vi "niFpgaBFGroupLastEven.vi"(5 "bf data in":T1 {"x_r" format="%.16g"; "x_i" format="%.16g"; "y_r" format="%.16g"; "y_i" format="%.16g"}, 7 "stage switch in":bool, 9 "tf index in":fxp<+,7,7>) -> (6 "bf data out":T1 {"x_r" format="%.16g"; "x_i" format="%.16g"; "y_r" format="%.16g"; "y_i" format="%.16g"}, 8 "stage switch out":bool)   [LabVIEW 2017]
uses:
  <vilib>/rvi/FXPMathLib/basic elements/FxpDiscreteDelay/XNode/nifxpmath_DiscreteDelay.xnode
  <vilib>/rvi/Analysis/measure/FFT/supportingXNodes/permutation/XNode/niFpgaFFTPermutation.xnode
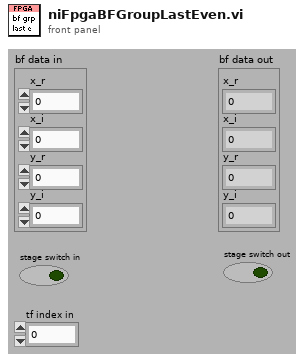
[diagram p1: front panel]
types:
  T1 = cluster{"x_r":fxp<+/-,16,1>, "x_i ":fxp<+/-,16,1>, "y_r ":fxp<+/-,16,1>, "y_i ":fxp<+/-,16,1>}
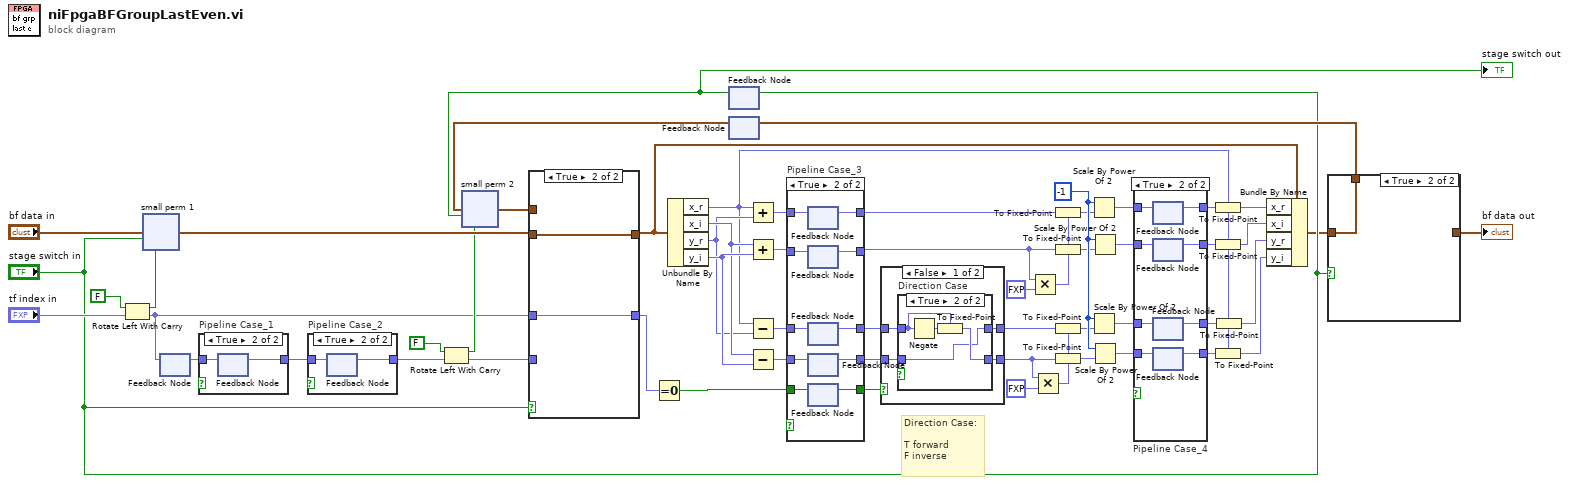
[diagram p0: block diagram]
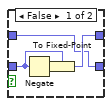
[diagram p6: hidden frame]
diagram:
  w31 = -1 ("n")
  # "Direction Case:\n\nT forward\nF inverse"
  n1 = Rotate Left With Carry(2:"tf index in", 3:FALSE ("carry")) -> (0:w34:fxp<+,7,7>, 1:w50:bool)
  n2 = xnode "small perm 1"("bf data in"="bf data in", "stage switch"="stage switch in", "perm switch"=w50) -> ("bf data out"=w49:T1)
  n3 = feedback-in #1(w34) -> ()
  n4 = feedback #1() -> (w11:fxp<+,7,7>)  [unwired: 1 in]
  n5 = case "Pipeline Case_1" shown="True" {
    selector: _ -> [_ _]
    tunnel: w11 -> [w59 w61]
    tunnel: [w59 w60] -> w2
    frame False {
    }
    frame True {
      n6 = feedback-in #2(w61) -> ()
      n7 = feedback #2() -> (w60:fxp<+,7,7>)  [unwired: 1 in]
    }
  }
  n8 = case "Pipeline Case_2" shown="True" {
    selector: _ -> [_ _]
    tunnel: w2 -> [w62 w64]
    tunnel: [w62 w63] -> w1
    frame False {
    }
    frame True {
      n9 = feedback-in #3(w64) -> ()
      n10 = feedback #3() -> (w63:fxp<+,7,7>)  [unwired: 1 in]
    }
  }
  n11 = Rotate Left With Carry(2:w1, 3:FALSE ("carry")) -> (0:w53:fxp<+,7,7>, 1:w48:bool)
  n12 = feedback-in #4("stage switch in") -> ()
  n13 = feedback #4() -> (w45:bool)  [unwired: 1 in]
  "stage switch out" <- w45
  n14 = feedback #5() -> (w47:T1)  [unwired: 1 in]
  n15 = xnode "small perm 2"("bf data in"=w47, "stage switch"=w45, "perm switch"=w48) -> ("bf data out"=w46:T1)
  n16 = case shown="True" "stage switch in" {
    tunnel: [w66 w68] -> w37
    tunnel: w49 -> [_ w68]
    tunnel: w46 -> [w66 _]
    tunnel: w53 -> [w65 _]
    tunnel: [w65 w67] -> w26
    tunnel: w34 -> [_ w67]
    frame False {
    }
    frame True {
    }
  }
  n17 = Equal To 0?(x=w26) -> (x = 0?=w13:bool)
  n18 = Unbundle By Name(w37) -> ("x_r"=w35:fxp<+/-,16,1>, "x_i"=w41:fxp<+/-,16,1>, "y_r"=w40:fxp<+/-,16,1>, "y_i"=w42:fxp<+/-,16,1>)
  n19 = Add(x=w35, y=w40) -> (x+y=w19:fxp<+/-,17,2>)
  n20 = Add(x=w41, y=w42) -> (x+y=w21:fxp<+/-,17,2>)
  n21 = Subtract(x=w35, y=w40) -> (x-y=w17:fxp<+/-,17,2>)
  n22 = Subtract(x=w41, y=w42) -> (x-y=w15:fxp<+/-,17,2>)
  n23 = case "Pipeline Case_3" shown="True" {
    selector: _ -> [_ _]
    tunnel: w21 -> [w72 w83]
    tunnel: [w72 w82] -> w20
    tunnel: w19 -> [w73 w81]
    tunnel: [w73 w80] -> w18
    tunnel: w17 -> [w71 w79]
    tunnel: [w71 w78] -> w16
    tunnel: w15 -> [w70 w77]
    tunnel: [w70 w76] -> w14
    tunnel: w13 -> [w69 w75]
    tunnel: [w69 w74] -> w12
    frame False {
    }
    frame True {
      n24 = feedback-in #6(w81) -> ()
      n25 = feedback #6() -> (w80:fxp<+/-,17,2>)  [unwired: 1 in]
      n26 = feedback-in #7(w83) -> ()
      n27 = feedback #7() -> (w82:fxp<+/-,17,2>)  [unwired: 1 in]
      n28 = feedback-in #8(w79) -> ()
      n29 = feedback #8() -> (w78:fxp<+/-,17,2>)  [unwired: 1 in]
      n30 = feedback-in #9(w77) -> ()
      n31 = feedback #9() -> (w76:fxp<+/-,17,2>)  [unwired: 1 in]
      n32 = feedback-in #10(w75) -> ()
      n33 = feedback #10() -> (w74:bool)  [unwired: 1 in]
    }
  }
  n34 = case shown="False" w12 {
    tunnel: w16 -> [w87 w97]
    tunnel: [w84 w97] -> w30
    tunnel: w14 -> [w85 w96]
    tunnel: [w86 w96] -> w24
    frame False {
      n35 = case "Direction Case" shown="True" {
        selector: _ -> [_ _]
        tunnel: w87 -> [w88 w94]
        tunnel: [w88 w93] -> w86
        tunnel: w85 -> [w90 w92]
        tunnel: [w89 w92] -> w84
        frame False {
          n36 = Negate(x=w90) -> (-x=w91:fxp<+/-,17,2>)
          n37 = To Fixed-Point(fixed-point type=w90, number=w91) -> (fixed-point=w89:fxp<+/-,17,2>)
        }
        frame True {
          n38 = Negate(x=w94) -> (-x=w95:fxp<+/-,17,2>)
          n39 = To Fixed-Point(fixed-point type=w94, number=w95) -> (fixed-point=w93:fxp<+/-,17,2>)
        }
      }
    }
    frame True {
    }
  }
  n40 = Multiply(x=w20, y=fxp<+,2,1> 0.0 ("x")) -> (x*y=w23:fxp<+/-,18,2>)
  n41 = Multiply(x=w24, y=fxp<+,2,1> 0.0 ("x")) -> (x*y=w22:fxp<+/-,18,2>)
  n42 = To Fixed-Point(fixed-point type=w23, number=w18) -> (fixed-point=w27:fxp<+/-,18,2>)
  n43 = To Fixed-Point(fixed-point type=w23, number=w20) -> (fixed-point=w28:fxp<+/-,18,2>)
  n44 = To Fixed-Point(fixed-point type=w22, number=w30) -> (fixed-point=w29:fxp<+/-,18,2>)
  n45 = To Fixed-Point(fixed-point type=w22, number=w24) -> (fixed-point=w32:fxp<+/-,18,2>)
  n46 = Scale By Power Of 2(n=w31, x=w27) -> (x*2^n=w10:fxp<+/-,18,2>)
  n47 = Scale By Power Of 2(n=w31, x=w29) -> (x*2^n=w8:fxp<+/-,18,2>)
  n48 = Scale By Power Of 2(n=w31, x=w28) -> (x*2^n=w9:fxp<+/-,18,2>)
  n49 = Scale By Power Of 2(n=w31, x=w32) -> (x*2^n=w7:fxp<+/-,18,2>)
  n50 = case "Pipeline Case_4" shown="True" {
    selector: _ -> [_ _]
    tunnel: w9 -> [w100 w109]
    tunnel: [w100 w108] -> w4
    tunnel: w10 -> [w101 w107]
    tunnel: [w101 w106] -> w3
    tunnel: w8 -> [w99 w105]
    tunnel: [w99 w104] -> w5
    tunnel: w7 -> [w98 w103]
    tunnel: [w98 w102] -> w6
    frame False {
    }
    frame True {
      n51 = feedback-in #11(w107) -> ()
      n52 = feedback #11() -> (w106:fxp<+/-,18,2>)  [unwired: 1 in]
      n53 = feedback-in #12(w109) -> ()
      n54 = feedback #12() -> (w108:fxp<+/-,18,2>)  [unwired: 1 in]
      n55 = feedback-in #13(w105) -> ()
      n56 = feedback #13() -> (w104:fxp<+/-,18,2>)  [unwired: 1 in]
      n57 = feedback-in #14(w103) -> ()
      n58 = feedback #14() -> (w102:fxp<+/-,18,2>)  [unwired: 1 in]
    }
  }
  n59 = To Fixed-Point(fixed-point type=w35, number=w3) -> (fixed-point=w39:fxp<+/-,16,1>)
  n60 = To Fixed-Point(fixed-point type=w35, number=w4) -> (fixed-point=w38:fxp<+/-,16,1>)
  n61 = To Fixed-Point(fixed-point type=w35, number=w6) -> (fixed-point=w44:fxp<+/-,16,1>)
  n62 = To Fixed-Point(fixed-point type=w35, number=w5) -> (fixed-point=w43:fxp<+/-,16,1>)
  n63 = Bundle By Name(cluster=w37, "x_r"=w39, "x_i"=w38, "y_r"=w43, "y_i"=w44) -> (w36:T1)
  n64 = case shown="True" "stage switch in" {
    tunnel: [_ w111] -> w58
    tunnel: w36 -> [w110 w111]
    tunnel: [w110 _] -> w57
    frame False {
    }
    frame True {
    }
  }
  "bf data out" <- w57
  n65 = feedback-in #5(w58) -> ()
